vi "Calculate Plot Range.vi"(8 "error in (no error)":errorcluster, 9 "Coordinates System":enum16{"Cartesian", "Cylindrical", "Spherical"}(ring), 10 "3D Stem Datatype.lvclass in":refnum<class "3D Stem Datatype.lvclass">, 11 "Plot Representation In":T1) -> (0 "error out":errorcluster, 2 "3D Stem Datatype.lvclass out":refnum<class "3D Stem Datatype.lvclass">, 3 "Plot Representation Out":T1)   [LabVIEW 2017, in "3D Stem Datatype.lvclass"]
uses:
  <vilib>/Math Plots/3D Math Plots/3D Stem/3D Stem Datatype/3D Stem Datatype.lvclass
  <vilib>/Math Plots/3D Math Plots/3D Plot/3D Plot/Typedef/Plot Representation.ctl
  <vilib>/Math Plots/3D Math Plots/3D Plot/3D Plot/Typedef/Range Clusters.ctl
  <vilib>/Math Plots/3D Math Plots/3D Plot/3D Plot/Typedef/Mesh Data.ctl
  <vilib>/Math Plots/3D Math Plots/3D Plot/3D Plot Datatype/3D Plot Datatype.lvclass
  <vilib>/Math Plots/3D Math Plots/3D Plot/3D Plot/3D Plot.lvclass
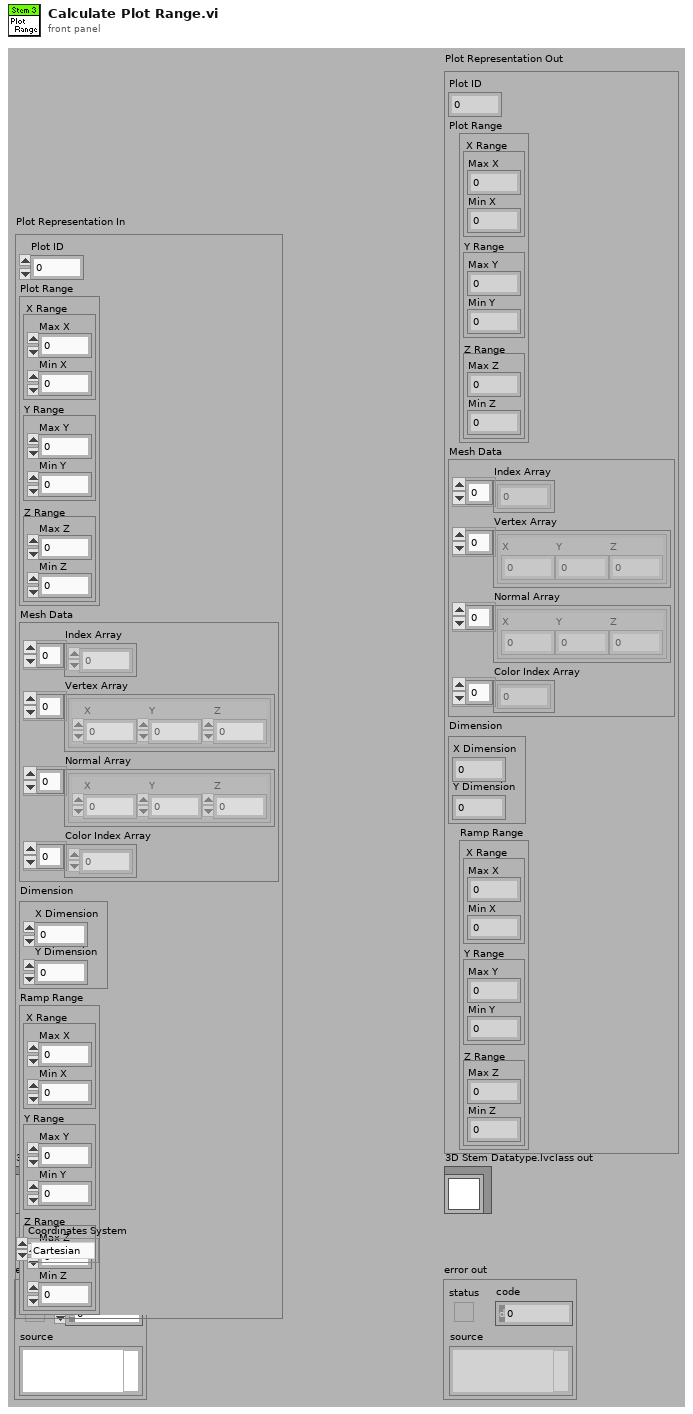
[diagram p1: front panel]
types:
  T1 = typedef "3D Plot.lvclass/Plot Representation.ctl" = cluster{"Plot ID":i32, "Plot Range":T2, "Mesh Data":T3, "Dimension":cluster{"X Dimension":i32, "Y Dimension":i32}, "Ramp Range":T2}
  T2 = typedef "3D Plot.lvclass/Range Clusters.ctl" = cluster{"X Range":cluster{"Max X":sgl, "Min X":sgl}, "Y Range":cluster{"Max Y":sgl, "Min Y":sgl}, "Z Range":cluster{"Max Z":sgl, "Min Z":sgl}}
  T3 = typedef "3D Plot.lvclass/Mesh Data.ctl" = cluster{"Index Array":u32[], "Vertex Array":cluster{"X":sgl, "Y":sgl, "Z":sgl}[], "Normal Array":cluster{"X":sgl, "Y":sgl, "Z":sgl}[], "Color Index Array":i32[]}
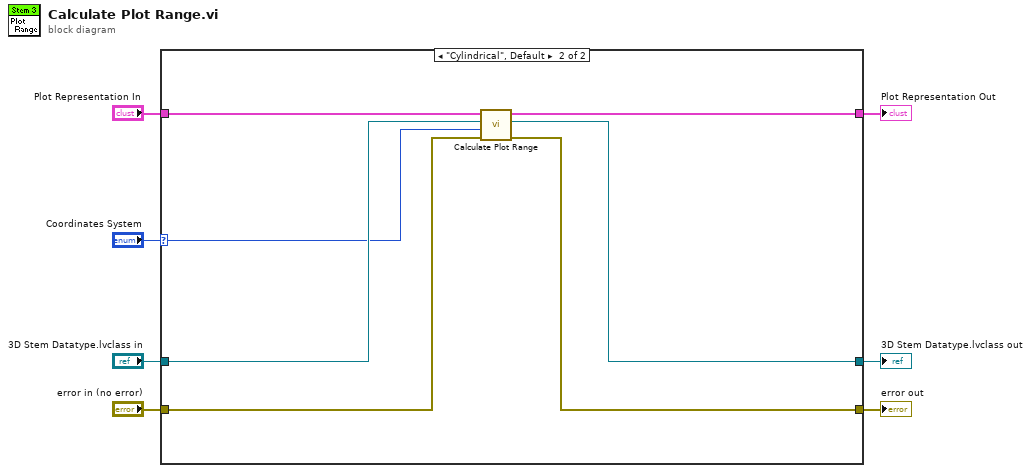
[diagram p0: block diagram]
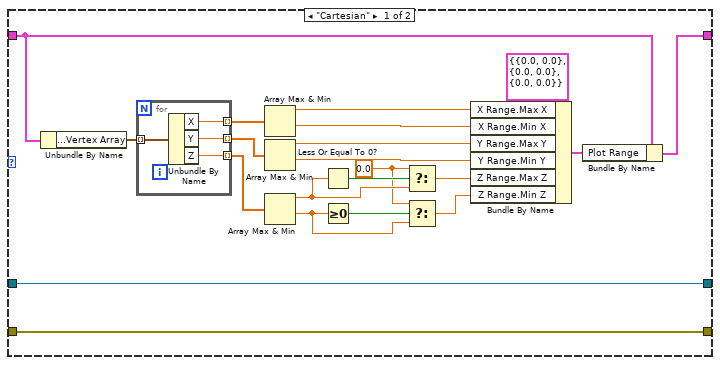
[diagram p2: hidden frame]
diagram:
  n1 = case shown="\"Cylindrical\", Default" "Coordinates System" {
    selector: "Coordinates System" -> [_ w35]
    tunnel: "3D Stem Datatype.lvclass in" -> [w23 w37]
    tunnel: [w23 w36] -> w6
    tunnel: [w21 w38] -> w5
    tunnel: "Plot Representation In" -> [w12 w39]
    tunnel: "error in (no error)" -> [w13 w34]
    tunnel: [w13 w33] -> w1
    frame "Cartesian" {
      w15 = sgl 0.0 ("t")
      n2 = Unbundle By Name(w12) -> ("Mesh Data.Vertex Array"=w11:cluster{"X":sgl, "Y":sgl, "Z":sgl}[])
      n3 = for {
        tunnel: w11 -> [w32] mode=indexing
        tunnel: [w31] -> w10 mode=indexing
        tunnel: [w30] -> w9 mode=indexing
        tunnel: [w29] -> w8 mode=indexing
        n4 = Unbundle By Name(w32) -> ("X"=w31:sgl, "Y"=w30:sgl, "Z"=w29:sgl)
      }
      n5 = Array Max & Min(array=w10) -> (max value=w27:sgl, min value=w26:sgl)  [unwired: 2 out]
      n6 = Array Max & Min(array=w9) -> (max value=w25:sgl, min value=w24:sgl)  [unwired: 2 out]
      n7 = Array Max & Min(array=w8) -> (max value=w16:sgl, min value=w14:sgl)  [unwired: 2 out]
      n8 = Less Or Equal To 0?(x=w16) -> (x <= 0?=w20:bool)
      n9 = Greater Or Equal To 0?(x=w14) -> (x >= 0?=w19:bool)
      n10 = Select(t=w15, s=w20, f=w16) -> (s? t:f=w18:sgl)
      n11 = Select(t=w15, s=w19, f=w14) -> (s? t:f=w17:sgl)
      n12 = Bundle By Name(cluster=T2 {"X Range"={"Max X"=0.0, "Min X"=0.0}, "Y Range"={"Max Y"=0.0, "Min Y"=0.0}, "Z Range"={"Max Z"=0.0, "Min Z"=0.0}} ("This Range Min/Max Out"), "X Range.Max X"=w27, "X Range.Min X"=w26, "Y Range.Max Y"=w25, "Y Range.Min Y"=w24, "Z Range.Max Z"=w18, "Z Range.Min Z"=w17) -> (w22:T2)
      n13 = Bundle By Name(cluster=w12, "Plot Range"=w22) -> (w21:T1)
    }
    frame "Cylindrical", Default {
      n14 = call-parent "Calculate Plot Range.vi"("error in (no error)"=w34, "Coordinates System"=w35, "3D Plot Datatype.lvclass in"=w37, "Plot Representation In"=w39) -> ("error out"=w33:errorcluster, "3D Plot Datatype.lvclass out"=w36:refnum<class "3D Stem Datatype.lvclass">, "Plot Representation Out"=w38:T1)  [unwired: 5 out]
    }
  }
  "error out" <- w1
  "3D Stem Datatype.lvclass out" <- w6
  "Plot Representation Out" <- w5
